vi "Problem 9.vi"() -> (0 "a*b*c":dbl format="%#_6f", 1 "c":dbl, 2 "b":i32, 3 "a":i32)   [LabVIEW 2013, in "Problem 9.lvlib"]
uses:
  Problem 9.lvlib
panel:
  out "a+b+c":dbl
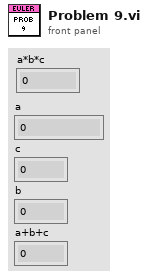
[diagram p1: front panel]
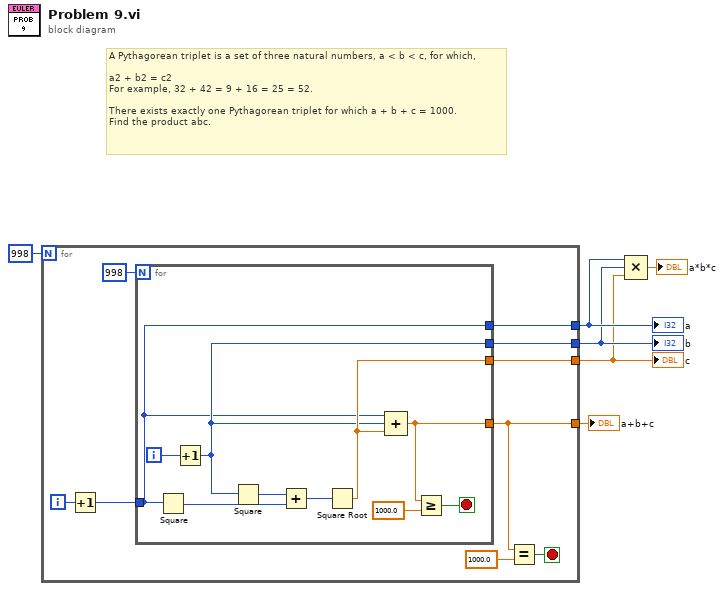
[diagram p0: block diagram]
diagram:
  # "A Pythagorean triplet is a set of three natural numbers, a < b < c, for which,\n\na2 + b2 = c2\nFor example, 32 + 42 = 9 + 16 = 25 = 52.\n\nThere exists exactly one Pythagorean triplet for which a + b + c = 1000.\nFind the product abc."
  n1 = for {
    N: 998 -> [_]
    tunnel: [w10] -> w4
    tunnel: [w9] -> w3
    tunnel: [w8] -> w2
    tunnel: [w7] -> w5
    i -> [w15]
    stop <- w12 stop-if-true
    n2 = Increment(x=w15) -> (x+1=w14:i32)
    n3 = for {
      N: 998 -> [_]
      tunnel: w14 -> [w16]
      tunnel: [w21] -> w7
      tunnel: [w16] -> w10
      tunnel: [w17] -> w9
      tunnel: [w19] -> w8
      i -> [w25]
      stop <- w23 stop-if-true
      n4 = Square(x=w16) -> (x^2=w18:i32)
      n5 = Increment(x=w25) -> (x+1=w17:i32)
      n6 = Square(x=w17) -> (x^2=w20:i32)
      n7 = Add(x=w20, y=w18) -> (x+y=w24:i32)
      n8 = Square Root(x=w24) -> (sqrt(x)=w19:dbl)
      n9 = Compound Arithmetic op=ADD(w16, w17, w19) -> (w21:dbl)
      n10 = Greater Or Equal?(x=w21, y=1000.0) -> (x >= y?=w23:bool)
    }
    n11 = Equal?(x=w7, y=1000.0) -> (x = y?=w12:bool)
  }
  "a" <- w4
  "b" <- w3
  "c" <- w2
  "a+b+c" <- w5
  n12 = Compound Arithmetic op=MULTIPLY(w4, w3, w2) -> (→"a*b*c":dbl)
